vi "Convert dec to hex.vi"(11 "P.u. Voltage":dbl) -> (3 "Numeric":dbl)   [LabVIEW 2022 SP3]
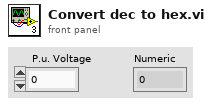
[diagram p1: front panel]
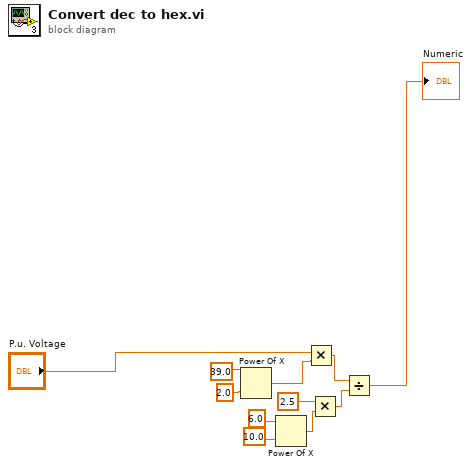
[diagram p0: block diagram]
diagram:
  n1 = Power Of X(1:2.0 ("x"), 2:39.0 ("y")) -> (0:w5:dbl)
  n2 = Power Of X(1:10.0 ("x"), 2:6.0 ("y")) -> (0:w7:dbl)
  n3 = Multiply(x="P.u. Voltage", y=w5) -> (x*y=w8:dbl)
  n4 = Multiply(x=2.5, y=w7) -> (x*y=w9:dbl)
  n5 = Divide(x=w8, y=w9) -> (x/y=→"Numeric":dbl)
